vi "ET2604 - Check Temperature and Humidity.vi"(5 "error in (no error)":errorcluster, 6 "VISA input":refnum<visa-resource-name>, 7 "Error de Humedad":sgl, 8 "Humedad Fijada":sgl, 9 "Error de Temperatura":sgl, 10 "Temperatura Fijada":sgl) -> (0 "error out":errorcluster, 1 "Humedad Medida":sgl, 2 "Temperatura Medida":sgl, 3 "VISA output":refnum<visa-resource-name>, 4 "¿En Rango?":bool)   [LabVIEW 2017]
doc: "Devuelve TRUE si las variables estan dentro de lo fijado +/- error. De estar fuera de rango, devuelve FALSE"
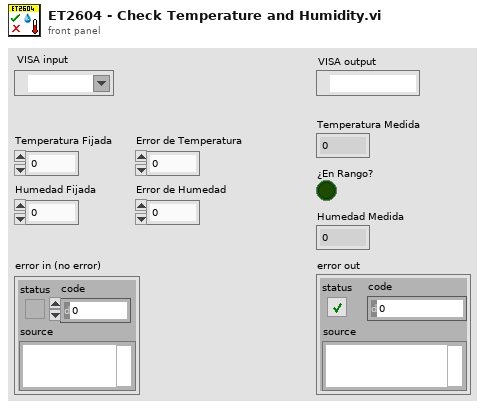
[diagram p1: front panel]
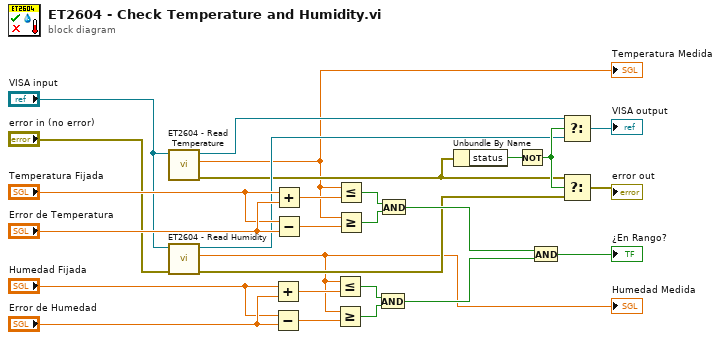
[diagram p0: block diagram]
diagram:
  n1 = call "ET2604 - Read Temperature.vi"("VISA resource name"="VISA input") -> ("error out"=w6:errorcluster, "Data"=w2:sgl, "VISA resource name out"=w9:refnum<visa-resource-name>)  [unwired: 7 in]
  "Temperatura Medida" <- w2
  n2 = call "ET2604 - Read Humidity.vi"("error in (no error)"="error in (no error)", "VISA resource name"="VISA input") -> ("error out"=w5:errorcluster, "Data"=w1:sgl, "VISA resource name out"=w8:refnum<visa-resource-name>)  [unwired: 7 in]
  "Humedad Medida" <- w1
  n3 = Add(x="Humedad Fijada", y="Error de Humedad") -> (x+y=w25:sgl)
  n4 = Subtract(x="Humedad Fijada", y="Error de Humedad") -> (x-y=w24:sgl)
  n5 = Add(x="Temperatura Fijada", y="Error de Temperatura") -> (x+y=w22:sgl)
  n6 = Subtract(x="Temperatura Fijada", y="Error de Temperatura") -> (x-y=w23:sgl)
  n7 = Less Or Equal?(x=w1, y=w25) -> (x <= y?=w27:bool)
  n8 = Greater Or Equal?(x=w1, y=w24) -> (x >= y?=w26:bool)
  n9 = Less Or Equal?(x=w2, y=w22) -> (x <= y?=w20:bool)
  n10 = Greater Or Equal?(x=w2, y=w23) -> (x >= y?=w21:bool)
  n11 = And(x=w27, y=w26) -> (x .and. y?=w18:bool)
  n12 = And(x=w20, y=w21) -> (x .and. y?=w19:bool)
  n13 = Unbundle By Name(w6) -> ("status"=w7:bool)
  n14 = Not(x=w7) -> (.not. x?=w10:bool)
  n15 = And(x=w19, y=w18) -> (x .and. y?=→"¿En Rango?":bool)
  n16 = Select(t=w9, s=w10, f=w8) -> (s? t:f=→"VISA output":refnum<visa-resource-name>)
  n17 = Select(t=w6, s=w10, f=w5) -> (s? t:f=→"error out":errorcluster)
